vi "Send and Return Events.vi"(8 "error in (no error)":errorcluster, 10 "Timeout (ms)":i32, 11 "Message Enqueuer":refnum<class "Message Enqueuer.lvclass">) -> (0 "error out":errorcluster, 1 "Timed Out?":bool, 2 "Event Cluster Out":T1, 3 "Message Enqueuer out":refnum<class "Message Enqueuer.lvclass">)   [LabVIEW 2015, in "Broadcast Actor.lvlib" / "Return Events Msg.lvclass"]
uses:
  Return Events Msg.lvclass
  Broadcast Actor.lvclass
  <vilib>/ActorFramework/Message Enqueuer/Message Enqueuer.lvclass
  Broadcast Actor/Type Defs/Events Type Def.ctl
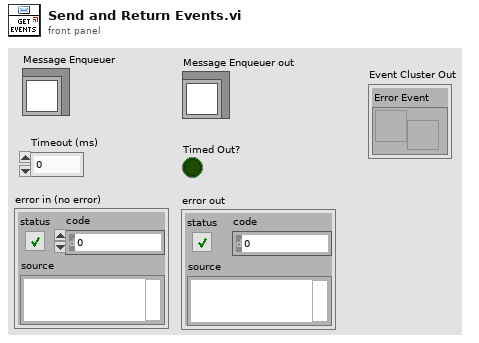
[diagram p1: front panel]
types:
  T1 = typedef "Broadcast Actor.lvlib/Broadcast Actor.lvclass/Events Type Def.ctl" = cluster{"Error Event":refnum<user-event>}
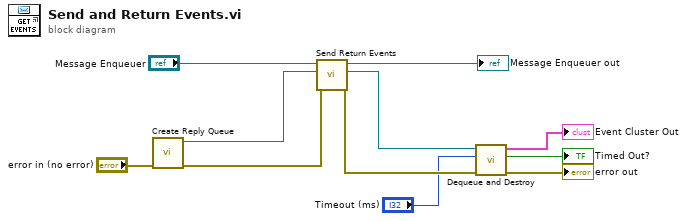
[diagram p0: block diagram]
diagram:
  n1 = call "Create Reply Queue.vi"("error in (no error)"="error in (no error)") -> ("error out"=w9:errorcluster, "Reply Queue Out"=w10:refnum<queue>)  [unwired: 9 in]
  n2 = call "Send Return Events.vi"("error in (no error)"=w9, "Reply Queue In"=w10, "Message Enqueuer"="Message Enqueuer") -> ("error out"=w8:errorcluster, "Reply Queue Out"=w11:refnum<queue>, "Message Enqueuer out"=→"Message Enqueuer out":refnum<class "Message Enqueuer.lvclass">)  [unwired: 6 in]
  n3 = call "Dequeue and Destroy.vi"("error in (no error)"=w8, "Timeout (ms)"="Timeout (ms)", "Reply Queue In"=w11) -> ("error out"=→"error out":errorcluster, "Timed Out?"=→"Timed Out?":bool, "Event Cluster Out"=→"Event Cluster Out":T1)  [unwired: 6 in]
